vi "toString.vi"(7 "UTC? (F)":bool, 9 "Timestamp (now)":timestamp, 11 "DateTime.ISO8601 in":refnum<class "DateTime.ISO8601.lvclass">) -> (1 "DateTime String":string, 3 "DateTime.ISO8601 out":refnum<class "DateTime.ISO8601.lvclass">)   [LabVIEW 2018, in "DateTime.ISO8601.lvclass"]
uses:
  DateTime.ISO8601.lvclass
  DateTime.ISO8601.lvclass/DateTime.ISO8601.ctl
  Timestamp to ISO8601 Day.vi
  isLeapYear (timestamp).vi
  Timestamp to ISO8601 Year.vi
  isLeapYear (integer).vi
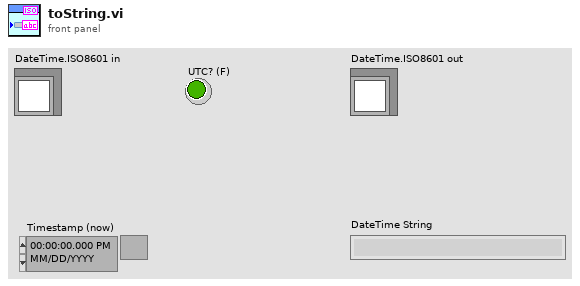
[diagram p1: front panel]
types:
  T1 = typedef "ISO8601 Date Formats.ctl" = enum16{"UTC Date-Time", "Date", "Calendar Month", "Week", "Week-Day", "Month-Day", "Ordinal Date"}
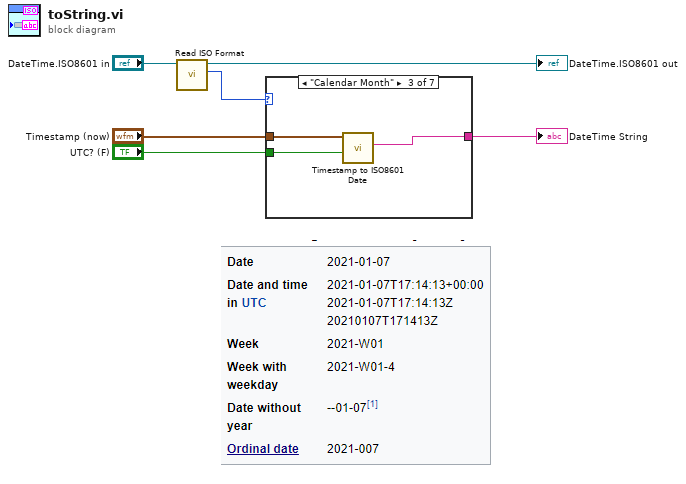
[diagram p0: block diagram]
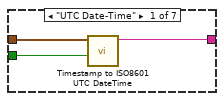
[diagram p2: hidden frame]
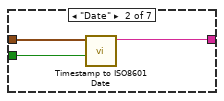
[diagram p3: hidden frame]
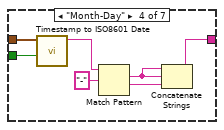
[diagram p4: hidden frame]
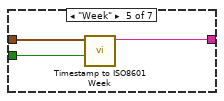
[diagram p5: hidden frame]
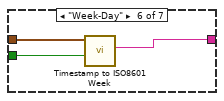
[diagram p6: hidden frame]
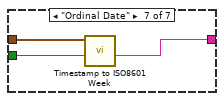
[diagram p7: hidden frame]
diagram:
  n1 = call "Read ISO Format.vi"("DateTime.ISO8601 in"="DateTime.ISO8601 in") -> ("ISO Format"=w1:T1, "DateTime.ISO8601 out"=→"DateTime.ISO8601 out":refnum<class "DateTime.ISO8601.lvclass">)  [unwired: 9 in]
  n2 = case shown="\"Calendar Month\"" w1 {
    tunnel: "Timestamp (now)" -> [w9 w12 w15 w22 w25 w28 w31]
    tunnel: [w8 w10 w13 w17 w23 w26 w29] -> w5
    tunnel: "UTC? (F)" -> [w7 w11 w14 w21 w24 w27 w30]
    frame "UTC Date-Time" {
      n3 = call "Timestamp to ISO8601 UTC DateTime.vi"("UTC? (F)"=w7, "Timestamp (now)"=w9) -> ("ISO8601 UTC DateTime"=w8:string)  [unwired: 9 in]
    }
    frame "Date" {
      n4 = call "Timestamp to ISO8601 Date.vi"("UTC? (F)"=w11, "Timestamp (now)"=w12) -> ("ISO8601 Date"=w10:string)  [unwired: 8 in, 1 out]
    }
    frame "Calendar Month" {
      n5 = call "Timestamp to ISO8601 Date.vi"("UTC? (F)"=w14, "Timestamp (now)"=w15) -> ("ISO8601 Calendar Month"=w13:string)  [unwired: 8 in, 1 out]
    }
    frame "Month-Day" {
      n6 = call "Timestamp to ISO8601 Date.vi"("UTC? (F)"=w21, "Timestamp (now)"=w22) -> ("ISO8601 Date"=w18:string)  [unwired: 8 in, 1 out]
      n7 = Match Pattern(string=w18, regular expression="-") -> (match substring=w16:string, after substring=w19:string)  [unwired: 1 in, 2 out]
      n8 = Concatenate Strings(w16, w16, w19) -> (w17:string)
    }
    frame "Week" {
      n9 = call "Timestamp to ISO8601 Week.vi"("UTC? (F)"=w24, "Timestamp (now)"=w25) -> ("ISO8601 Week"=w23:string)  [unwired: 7 in, 2 out]
    }
    frame "Week-Day" {
      n10 = call "Timestamp to ISO8601 Week.vi"("UTC? (F)"=w27, "Timestamp (now)"=w28) -> ("ISO8601 Weekday"=w26:string)  [unwired: 7 in, 2 out]
    }
    frame "Ordinal Date" {
      n11 = call "Timestamp to ISO8601 Week.vi"("UTC? (F)"=w30, "Timestamp (now)"=w31) -> ("ISO8601 Ordinal Date"=w29:string)  [unwired: 7 in, 2 out]
    }
  }
  "DateTime String" <- w5
